vi "Get Subsystem Color.vi"(11 "VI in":refnum<vi>) -> (3 "Color Box":u32(colorbox))   [LabVIEW 2025]
uses:
  <vilib>/LabVIEW Icon API/lv_icon/Classes/Icon/Icon.lvclass
  <vilib>/LabVIEW Icon API/lv_icon/Classes/Layer/Layer.lvclass
  <vilib>/LabVIEW Icon API/LabVIEW Icon API.lvlib
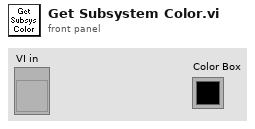
[diagram p1: front panel]
types:
  T1 = cluster{"left":i16, "top":i16, "right":i16, "bottom":i16}
  T2 = typedef "Layer.ctl" = cluster{"LayerIcon":picture, "LayerName":string, "Opacity":u8, "Visibility?":bool}
  T3 = typedef "imagedata.ctl" = cluster{"image type":i32, "image depth":i32, "image":u8[], "mask":u8[], "colors":u32[], "Rectangle":cluster{"left":i16, "top":i16, "right":i16, "bottom":i16}}
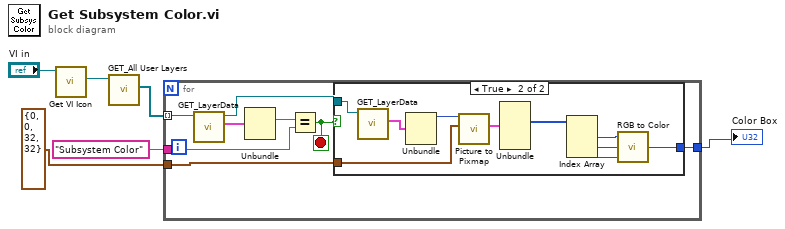
[diagram p0: block diagram]
diagram:
  n1 = call <vilib>:"Get VI Icon.vi"("VI Refnum in"="VI in") -> ("Icon"=w2:refnum<class "Icon.lvclass">)  [unwired: 8 in, 2 out]
  n2 = call-dynamic "GET_All User Layers.vi"("Icon.lvclass in"=w2) -> ("User Layer"=w4:refnum<class "Layer.lvclass">[])  [unwired: 8 in, 2 out]
  n3 = for {
    tunnel: w4 -> [w11] mode=indexing
    tunnel: "Subsystem Color" ("Layer name") -> [w13]
    tunnel: T1 {"left"=0, "top"=0, "right"=32, "bottom"=32} ("rect") -> [w9]
    tunnel: [w8] -> w1
    stop <- w7 stop-if-true
    n4 = call-dynamic "GET_LayerData.vi"("Layer.lvclass in"=w11) -> ("Data"=w14:T2, "Layer.lvclass out"=w10:refnum<class "Layer.lvclass">)  [unwired: 6 in, 3 out]
    n5 = Unbundle(w14) -> ("LayerName"=w12:string)  [unwired: 3 out]
    n6 = Equal?(x=w12, y=w13) -> (x = y?=w7:bool)
    n7 = case shown="True" w7 {
      tunnel: w10 -> [_ w24]
      tunnel: w9 -> [_ w21]
      tunnel: [_ w15] -> w8
      frame False {
      }
      frame True {
        n8 = call-dynamic "GET_LayerData.vi"("Layer.lvclass in"=w24) -> ("Data"=w23:T2)  [unwired: 6 in, 4 out]
        n9 = Unbundle(w23) -> ("LayerIcon"=w22:picture)  [unwired: 3 out]
        n10 = call <vilib>:"Picture to Pixmap.vi"("rect"=w21, "picture"=w22) -> ("image data"=w20:T3)  [unwired: 8 in, 1 out]
        n11 = Unbundle(w20) -> ("image"=w19:u8[])  [unwired: 5 out]
        n12 = Index Array(array=w19) -> (element #1=w18:u8, element #2=w17:u8, element #3=w16:u8)  [unwired: 3 in]
        n13 = call <vilib>:"RGB to Color.vi"("B"=w16, "G"=w17, "R"=w18) -> ("Color"=w15:u32)
      }
    }
  }
  "Color Box" <- w1
